vi "Get check if at destination.vi"(8 "error in (no error)":errorcluster, 11 "focus in":refnum<class "focus.lvclass">) -> (0 "error out":errorcluster, 2 "check if at destination":bool, 3 "focus out":refnum<class "focus.lvclass">)   [LabVIEW 2012, in "focus.lvclass"]
uses:
  focus.lvclass
  focus.lvclass/focus.ctl
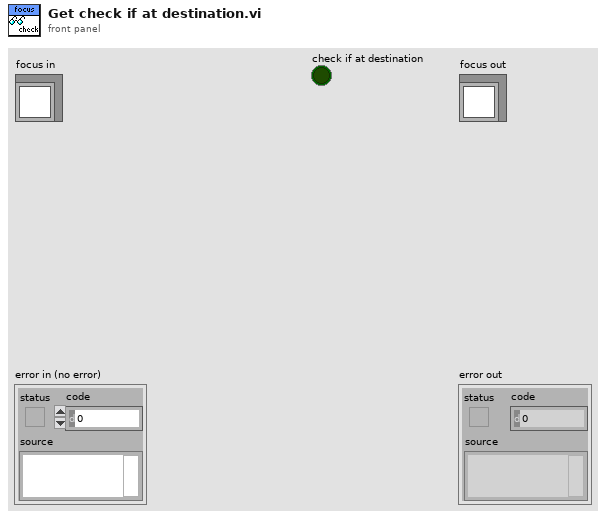
[diagram p1: front panel]
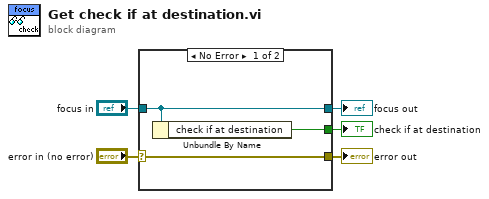
[diagram p0: block diagram]
diagram:
  n1 = case shown="No Error" "error in (no error)" {
    selector: "error in (no error)" -> [w8 w10]
    tunnel: [w8 w10] -> w4
    tunnel: [w7 w9] -> w2
    tunnel: "focus in" -> [w7 w9]
    tunnel: [w6 _] -> w1
    frame No Error {
      n2 = Unbundle By Name(w7) -> ("check if at destination"=w6:bool)
    }
    frame Error {
    }
  }
  "error out" <- w4
  "focus out" <- w2
  "check if at destination" <- w1
